vi "Export Data.vi"(8 "error in (no error)":cluster{"状态":bool, "代码":i32, "源":string} caption="错误输入（无错误）", 11 "图形数据":T1) -> (0 "error out":cluster{"状态":bool, "代码":i32, "源":string} caption="错误输出")   [LabVIEW 2013]
doc: "将当前显示的数据和分析结果导出至制表符分隔的文本文件，以便在其他电子表格应用程序中加载。"
uses:
  controls/Graph Data.ctl
  <vilib>/Utility/miscctls.llb/LVAnnotationListTypeDef.ctl
  <vilib>/Utility/miscctls.llb/LVCursorListTypeDef.ctl
  <vilib>/Waveform/WDTFileIO.llb/Export Waveforms To Spreadsheet File (1D).vi
panel:
  # "（向上滚动可查看大型数据簇）"
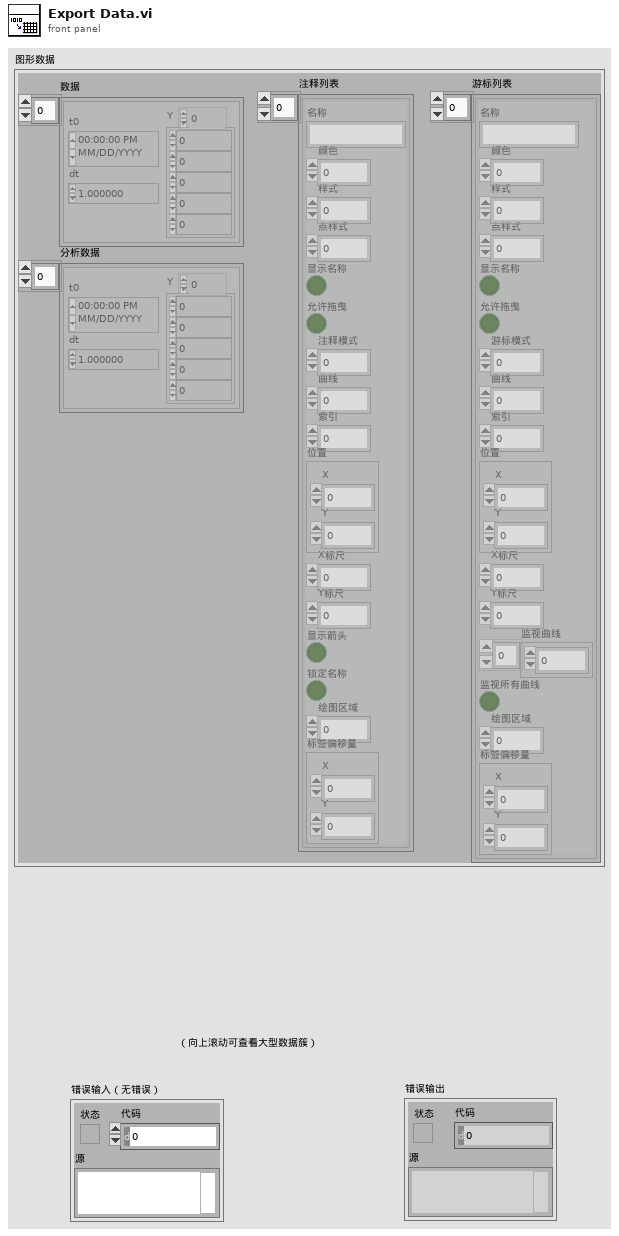
[diagram p1: front panel]
types:
  T1 = typedef "Graph Data.ctl" = cluster{"数据":waveform(dbl)[], "注释列表":T2, "游标列表":T3, "分析数据":waveform(dbl)[]}
  T2 = typedef "LVAnnotationListTypeDef.ctl" = cluster{"Name":string, "Color":u32, "Style":u8, "Point Style":u8, "Name Visible":bool, "Allow Drag":bool, "Annotation Mode":u32, "Plot":i32, "Index":i32, "Position":cluster{"X":dbl, "Y":dbl}, "X Scale":u32, "Y Scale":u32, "Show Arrow":bool, "Lock Name":bool, "Plot Area":i32, "Label Offset":cluster{"X":dbl, "Y":dbl}}[]
  T3 = typedef "LVCursorListTypeDef.ctl" = cluster{"Name":string, "Color":u32, "Style":u8, "Point Style":u8, "Name Visible":bool, "Allow Drag":bool, "Cursor Mode":u32, "Plot":i32, "Index":i32, "Position":cluster{"X":dbl, "Y":dbl}, "X Scale":u32, "Y Scale":u32, "Watch Plots":i32[], "Watch All Plots":bool, "Plot Area":i32, "Label Offset":cluster{"X":dbl, "Y":dbl}}[]
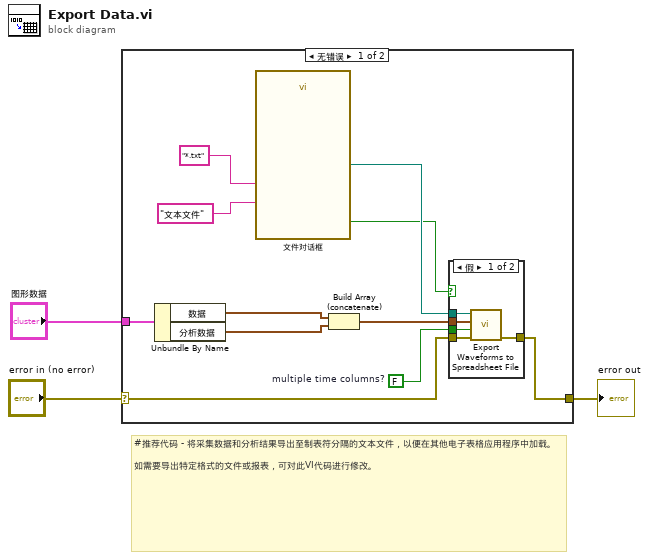
[diagram p0: block diagram]
diagram:
  # "#推荐代码 - 将采集数据和分析结果导出至制表符分隔的文本文件，以便在其他电子表格应用程序中加载。\n\n如需要导出特定格式的文件或报表，可对此VI代码进行修改。"
  n1 = case shown="无错误" "error in (no error)" {
    selector: "error in (no error)" -> [w12 w21]
    tunnel: "图形数据" -> [w14 _]
    tunnel: [w11 w21] -> w2
    frame No Error {
      w13 = FALSE  # multiple time columns?
      n2 = Unbundle By Name(w14) -> ("数据"=w10:waveform(dbl)[], "分析数据"=w9:waveform(dbl)[])
      n3 = call "文件对话框"("pattern (all files)"="*.txt", "pattern label"="文本文件" ("Text File")) -> ("selected path"=w7:path, "cancelled"=w4:bool)  [unwired: 10 in, 2 out]
      n4 = Build Array (concatenate)(w10, w9) -> (w8:waveform(dbl)[])
      n5 = case shown="假" w4 {
        tunnel: w13 -> [w19 _]
        tunnel: w12 -> [w18 w20]
        tunnel: [w17 w20] -> w11
        tunnel: w8 -> [w16 _]
        tunnel: w7 -> [w15 _]
        frame False {
          n6 = call-poly <vilib>:"Export Waveforms to Spreadsheet File.vi"("error in (no error)"=w18, "multiple time columns? (single:F)"=w19, "waveforms"=w16, "file path (dialog if empty)"=w15) -> ("error out"=w17:errorcluster)  [unwired: 6 in, 1 out]
        }
        frame True {
        }
      }
    }
    frame Error {
    }
  }
  "error out" <- w2
